vi "4155C Config QSCV params.vi"(0 "VISA session":refnum<visa-resource-name>, 1 "Drain Voltage":dbl min=-100.0 max=100.0 format="%.2f", 2 "Drain Compliance":dbl min=0.0 max=0.1 format="%^.2e", 3 "stop condition (free run:0)":u8(ring)=1 items=["continue at any (free run)", "stop at any abnorm", "stop at compliance"], 5 "HTIMe":dbl min=0.0 max=655.35 step=0.01 format="%.2f", 7 "DELay":dbl min=0.0 max=65.535 step=0.0001 format="%.2f", 9 "RANGe":dbl format="%.2f", 11 "error in (no error)":errorcluster, 12 "I-Int":dbl=0.1 min=0.02 max=2.0 format="%.2f", 13 "C-Int":dbl=0.1 min=0.04 max=400.0 format="%.2f") -> (4 "dup VISA resource name":refnum<visa-resource-name>, 15 "error out":errorcluster)   [LabVIEW 2016]
doc: "This VI configures the timing parameters of the measurement functions. The settings of this VI could be different from the actual instrument's settings due to limits imposed by other parameters inside the instrument. To check the actual values of integration time and number of power line cycles, run HP415xA Query Integration Time.vi."
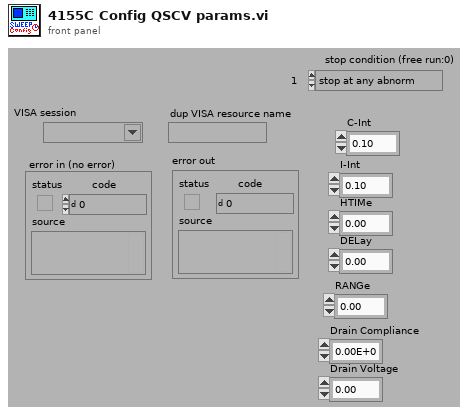
[diagram p1: front panel]
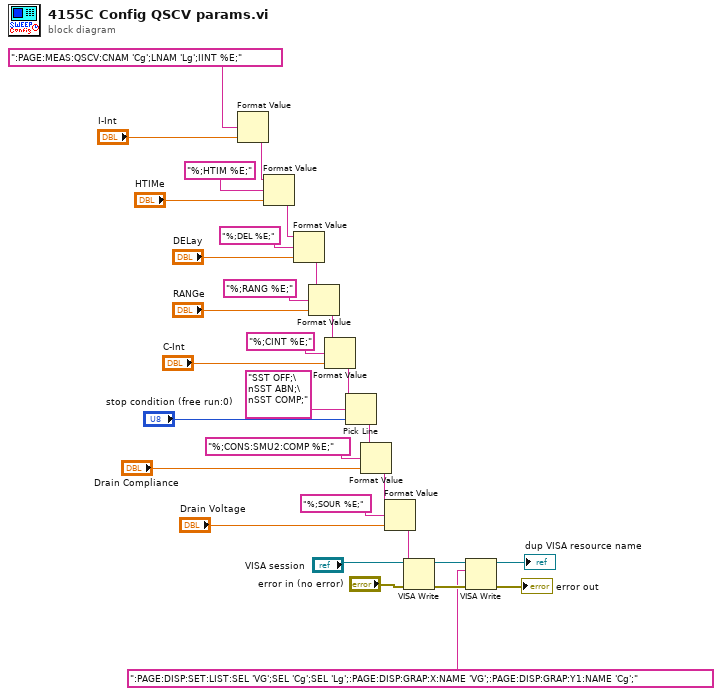
[diagram p0: block diagram]
diagram:
  n1 = Format Value(format string=":PAGE:MEAS:QSCV:CNAM 'Cg';LNAM 'Lg';IINT %E;", value (0)="I-Int") -> (output string=w25:string)  [unwired: 1 in]
  n2 = Format Value(string ("")=w25, format string="%;HTIM %E;", value (0)="HTIMe") -> (output string=w22:string)
  n3 = Format Value(string ("")=w22, format string="%;DEL %E;", value (0)="DELay") -> (output string=w18:string)
  n4 = Format Value(string ("")=w18, format string="%;RANG %E;", value (0)="RANGe") -> (output string=w14:string)
  n5 = Format Value(string ("")=w14, format string="%;CINT %E;", value (0)="C-Int") -> (output string=w8:string)
  n6 = Pick Line(string ("")=w8, multi-line string="SST OFF;\nSST ABN;\nSST COMP;", line index="stop condition (free run:0)") -> (output string=w7:string)
  n7 = Format Value(string ("")=w7, format string="%;CONS:SMU2:COMP %E;", value (0)="Drain Compliance") -> (output string=w11:string)
  n8 = Format Value(string ("")=w11, format string="%;SOUR %E;", value (0)="Drain Voltage") -> (output string=w6:string)
  n9 = VISA Write(VISA resource name="VISA session", write buffer=w6, error in (no error)="error in (no error)") -> (VISA resource name out=w2:refnum<visa-resource-name>, error out=w5:errorcluster)  [unwired: 1 out]
  n10 = VISA Write(VISA resource name=w2, write buffer=":PAGE:DISP:SET:LIST:SEL 'VG';SEL 'Cg';SEL 'Lg';:PAGE:DISP:GRAP:X:NAME 'VG';:PAGE:DISP:GRAP:Y1:NAME 'Cg';" ("write buffer (\"\")"), error in (no error)=w5) -> (VISA resource name out=→"dup VISA resource name":refnum<visa-resource-name>, error out=→"error out":errorcluster)  [unwired: 1 out]
